vi "usrp get rx antenna.vi"(8 "error in (no error)":errorcluster, 10 "chan":u64, 11 "h":u64) -> (0 "error out":errorcluster, 1 "ant_out out":string, 2 "function return":u32(ring), 3 "h 2":u64)   [LabVIEW 2023, in "uhd.lvlib"]
doc: "UHD_API uhd_error uhd_usrp_get_rx_antenna(\n uhd_usrp_handle h, size_t chan, char* ant_out, size_t strbuffer_len);"
uses:
  <userlib>/uhd/uhd.lvlib
  <userlib>/uhd/uhd.dll
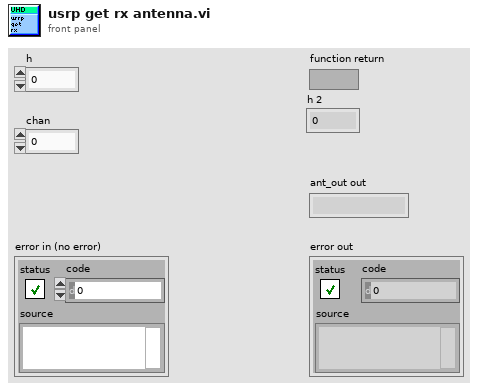
[diagram p1: front panel]
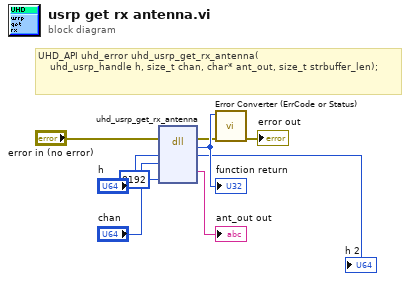
[diagram p0: block diagram]
diagram:
  # "UHD_API uhd_error uhd_usrp_get_rx_antenna(\n    uhd_usrp_handle h, size_t chan, char* ant_out, size_t strbuffer_len);"
  n1 = dll-call lib="C:/Program Files/National Instruments/LabVIEW 2023/user.lib/uhd/uhd.*" fn="uhd_usrp_get_rx_antenna"(error in="error in (no error)", "h"="h", "chan"="chan", "strbuffer_len"=u64 8192) -> (error out=w4:errorcluster, w9:u32, "h"=→"h 2":u64, "ant_out"=→"ant_out out":string)  [unwired: 5 in, 1 out]
  "function return" <- w9
  n2 = call <userlib>:"Error Converter (ErrCode or Status).vi"("error in (no error)"=w4, "error code"=w9) -> ("error out"=→"error out":errorcluster)  [unwired: 9 in]
